vi "Configure Gantry Head.vi"(7 "Config Folder":path, 8 "error in (no error)":errorcluster, 11 "WorkTable Class in":refnum<class "WorkTable Class.lvclass">) -> (0 "error out":errorcluster, 3 "WorkTable Class out":refnum<class "WorkTable Class.lvclass">)   [LabVIEW 2011, in "WorkTable Class.lvclass"]
uses:
  WorkTable Class.lvclass
  Type Definitions/Worktable_Gantry Head.ctl
  <vilib>/Utility/config.llb/Read Key (U32).vi
  <vilib>/Utility/config.llb/NI_LVConfig.lvlib
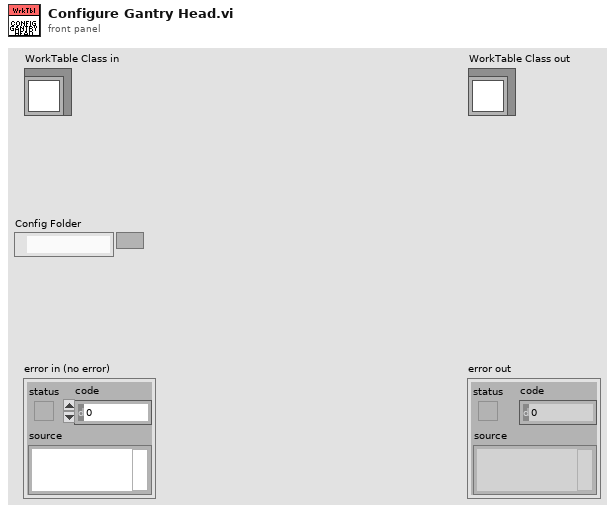
[diagram p1: front panel]
types:
  T1 = typedef "Worktable_Gantry Head.ctl" = cluster{"Current Tool":enum16{"None", "Grabber", "Picker", "Tool Setter"}, "Vacuum Channel Inner":u8, "Vacuum Channel Outer":u8, "Numeric":dbl}
  T2 = enum16{"None", "Grabber", "Picker", "Tool Setter"}
  T3 = typedef "NI_LVConfig.lvlib/Config Data RefNum.ctl" = refnum<k1>
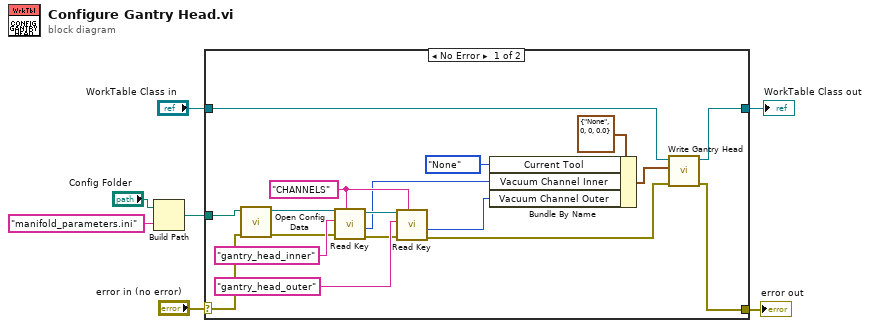
[diagram p0: block diagram]
diagram:
  n1 = Build Path(base path="Config Folder", name or relative path="manifold_parameters.ini") -> (appended path=w1:path)
  n2 = case shown="No Error" "error in (no error)" {
    selector: "error in (no error)" -> [w11 w27]
    tunnel: [w10 w27] -> w6
    tunnel: [w16 w26] -> w4
    tunnel: "WorkTable Class in" -> [w17 w26]
    tunnel: w1 -> [w25 _]
    frame No Error {
      w22 = "CHANNELS"
      n3 = call <vilib>:"Open Config Data.vi"("error in (no error)"=w11, "configuration file path"=w25) -> ("error out"=w19:errorcluster, "refnum"=w24:T3)  [unwired: 7 in, 1 out]
      n4 = call-poly <vilib>:"Read Key.vi"("section"=w22, "error in (no error)"=w19, "key"="gantry_head_inner", "refnum"=w24) -> ("error out"=w18:errorcluster, "value"=w14:u32, "refnum out"=w23:T3)  [unwired: 4 in, 1 out]
      n5 = call-poly <vilib>:"Read Key.vi"("section"=w22, "error in (no error)"=w18, "key"="gantry_head_outer", "refnum"=w23) -> ("error out"=w12:errorcluster, "value"=w13:u32)  [unwired: 4 in, 2 out]
      n6 = Bundle By Name(cluster=T1 {"Current Tool"=enum."None", "Vacuum Channel Inner"=0, "Vacuum Channel Outer"=0, "Numeric"=0.0} ("Gantry Head"), "Current Tool"=T2."None", "Vacuum Channel Inner"=w14, "Vacuum Channel Outer"=w13) -> (w8:T1)
      n7 = call-dynamic "Write Gantry Head.vi"("error in (no error)"=w12, "Gantry Head"=w8, "WorkTable Class in"=w17) -> ("error out"=w10:errorcluster, "WorkTable Class out"=w16:refnum<class "WorkTable Class.lvclass">)  [unwired: 7 in]
    }
    frame Error {
    }
  }
  "error out" <- w6
  "WorkTable Class out" <- w4
